vi "File_CleanClose.vi"(8 "error in (no error)":errorcluster, 11 "File in":refnum<class "File.lvclass">) -> (0 "error out":errorcluster, 3 "File out":refnum<class "File.lvclass">)   [LabVIEW 2023, in "File.lvclass"]
doc: "Closes the file and defragments the resulting TDMS file to preserve space."
uses:
  File.lvclass
  File.lvclass/File.ctl
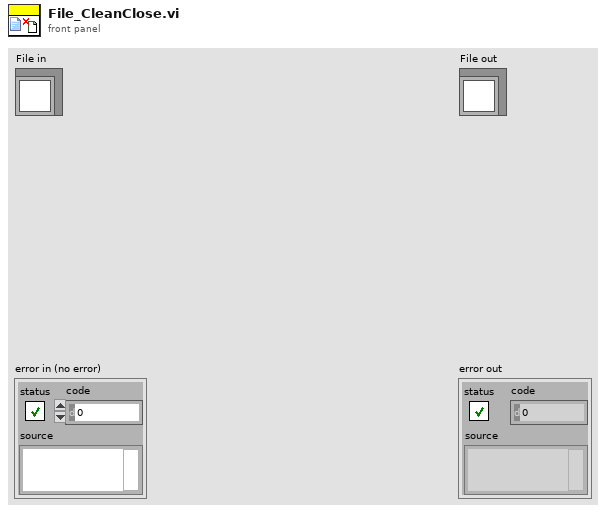
[diagram p1: front panel]
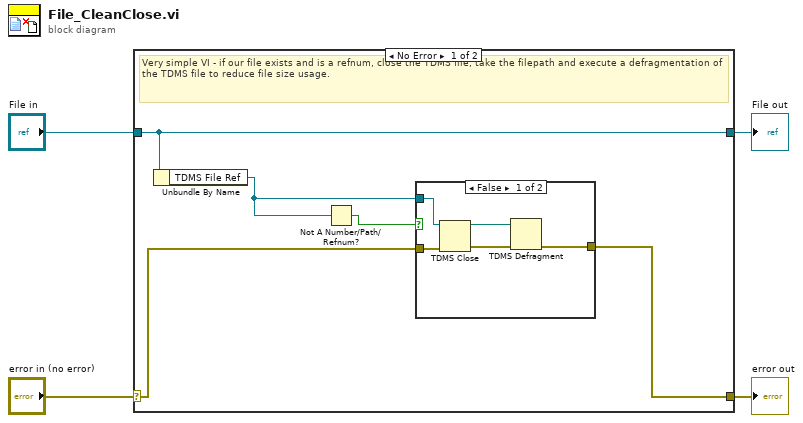
[diagram p0: block diagram]
diagram:
  n1 = case shown="No Error" "error in (no error)" {
    selector: "error in (no error)" -> [w9 w17]
    tunnel: [w8 w17] -> w3
    tunnel: [w7 w16] -> w1
    tunnel: "File in" -> [w7 w16]
    frame No Error {
      # "Very simple VI - if our file exists and is a refnum, close the TDMS file, take the filepath and execute a defragmentation of the TDMS file to reduce file size usage."
      n2 = Unbundle By Name(w7) -> ("TDMS File Ref"=w5:refnum<k34>)
      n3 = Not A Number/Path/Refnum?(number/path/refnum=w5) -> (NaN/Path/Refnum?=w6:bool)
      n4 = case shown="False" w6 {
        tunnel: w9 -> [w13 w15]
        tunnel: [w12 w15] -> w8
        tunnel: w5 -> [w10 _]
        frame False {
          n5 = TDMS Close(8:w13, 11:w10) -> (0:w14:errorcluster, 3:w11:path)
          n6 = TDMS Defragment(4:w14, 7:w11) -> (0:w12:errorcluster)
        }
        frame True {
        }
      }
    }
    frame Error {
    }
  }
  "error out" <- w3
  "File out" <- w1
